vi "CSTK_Icon_Creator_Dialong_CreateLogo_CoordsToArrayIndex.vi"(8 "错误输入（无错误）":errorcluster, 10 "Coords":T1, 11 "Array输入":refnum<vi>) -> (0 "错误输出":errorcluster, 2 "ArrayIndex":T1, 3 "Array输出":refnum<vi>)   [LabVIEW 2015, in "CSTK_Icon Creator.lvlib"]
uses:
  CSTK_Icon Creator.lvlib
  <vilib>/Utility/miscctls.llb/LVPoint32TypeDef.ctl
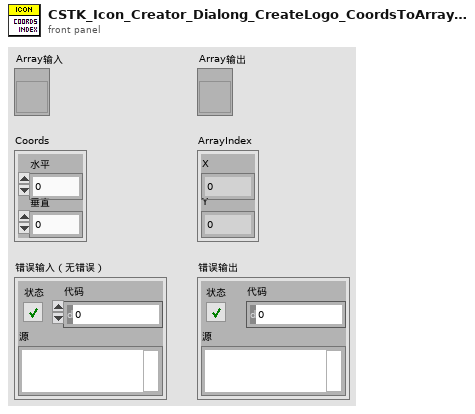
[diagram p1: front panel]
types:
  T1 = typedef "LVPoint32TypeDef.ctl" = cluster{"Horizontal":i32, "Vertical":i32}
  T2 = typedef "LVPositionTypeDef.ctl" = cluster{"Left":i32, "Top":i32}
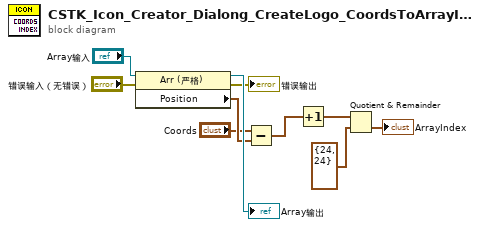
[diagram p0: block diagram]
diagram:
  n1 = property class="Arr (严格)"(reference="Array输入", error in="错误输入（无错误）") -> (reference out=→"Array输出":refnum<vi>, error out=→"错误输出":errorcluster, "Position"=w5:T2)
  n2 = Subtract(x="Coords", y=w5) -> (x-y=w6:T1)
  n3 = Increment(x=w6) -> (x+1=w7:T1)
  n4 = Quotient & Remainder(x=w7, y=T1 {"Horizontal"=24, "Vertical"=24}) -> (floor(x/y)=→"ArrayIndex":T1)  [unwired: 1 out]
